vi "Test Set PSU Z.vi"(8 "error in (no error)":errorcluster, 11 "Instrument.OxfordVRM in":refnum<class "Instrument.OxfordVRM.lvclass">) -> (0 "error out":errorcluster, 3 "Instrument.OxfordVRM out":refnum<class "Instrument.OxfordVRM.lvclass">)   [LabVIEW 2016, in "Instrument.OxfordVRM.lvclass"]
uses:
  Instrument.OxfordVRM.lvclass
  <vilib>/addons/_JKI Toolkits/Caraya/classes/Assert/Assert Not Error.vi
  <vilib>/addons/_JKI Toolkits/Caraya/classes/Assert/Assert Equal Value and Type_Variant.vi
  <vilib>/addons/_JKI Toolkits/Caraya/classes/Test/Test.lvclass
  <vilib>/addons/_JKI Toolkits/Caraya/classes/Assert/Assert.lvclass
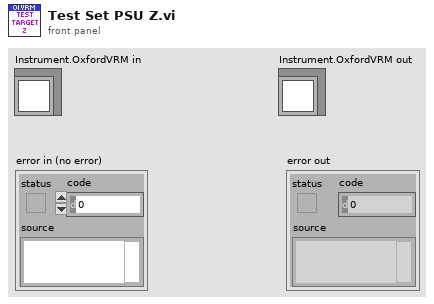
[diagram p1: front panel]
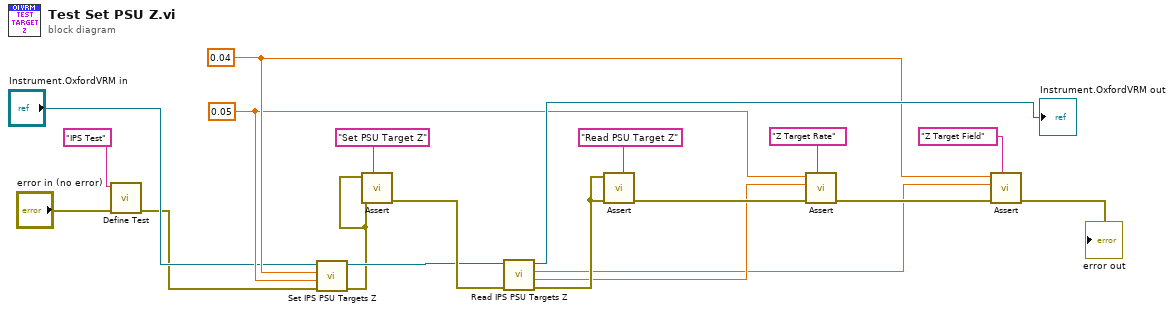
[diagram p0: block diagram]
diagram:
  w5 = 0.05 ("Target Field Rate (T/min)")
  w6 = 0.04 ("Target Field (T)")
  n1 = call <vilib>:"Define Test.vi"("error in (no error)"="error in (no error)", "Label (VI Title)"="IPS Test") -> ("error out"=w1:errorcluster)  [unwired: 9 in]
  n2 = call "Set IPS PSU Targets Z.vi"("error in (no error)"=w1, "Target Field Rate (T/min)"=w5, "Target Field (T)"=w6, "Instrument.OxfordVRM in"="Instrument.OxfordVRM in") -> ("error out"=w3:errorcluster, "Instrument.OxfordVRM out"=w4:refnum<class "Instrument.OxfordVRM.lvclass">)  [unwired: 5 in, 1 out]
  n3 = call-poly <vilib>:"Assert.vi"("Label"="Set PSU Target Z", "error in (no error)"=w3, "Not Error?"=w3) -> ("error out"=w18:errorcluster)  [unwired: 8 in]
  n4 = call "Read IPS PSU Targets Z.vi"("error in (no error)"=w18, "Instrument.OxfordVRM in"=w4) -> ("error out"=w17:errorcluster, "Target Field Rate (T/min)"=w11:dbl, "Target Field (T)"=w10:dbl, "Instrument.OxfordVRM out"=→"Instrument.OxfordVRM out":refnum<class "Instrument.OxfordVRM.lvclass">)  [unwired: 6 in]
  n5 = call-poly <vilib>:"Assert.vi"("Label"="Read PSU Target Z", "error in (no error)"=w17, "Not Error?"=w17) -> ("error out"=w14:errorcluster)  [unwired: 8 in]
  n6 = call-poly <vilib>:"Assert.vi"("Label"="Z Target Rate", "error in (no error)"=w14, "Y"=w11, "X"=w5) -> ("error out"=w13:errorcluster)  [unwired: 7 in]
  n7 = call-poly <vilib>:"Assert.vi"("Label"="Z Target Field", "error in (no error)"=w13, "Y"=w10, "X"=w6) -> ("error out"=→"error out":errorcluster)  [unwired: 7 in]
